vi "Motor Power Based on Vision.vi"() -> (1 "Right Motor Power":dbl, 3 "Left Motor Power":dbl)   [LabVIEW 2016]
uses:
  Robot Values.vi
  Vision Global.vi
  <vilib>/addons/control/pid/pid.llb/PID (DBL).vi
  <vilib>/addons/control/pid/NI_PID_pid.lvlib
panel:
  out "Vision Particles":dbl
  out "Done":bool
  in  "Vision PID Gains":T1={"proportional gain (Kc)"=0.2, "integral time (Ti, min)"=0.0, "derivative time (Td, min)"=0.0} {"derivative time (Td, min)" format="%.3f"; "integral time (Ti, min)" format="%.3f"; "proportional gain (Kc)" format="%.3f"}
  in  "Power Baseline":dbl=0.5
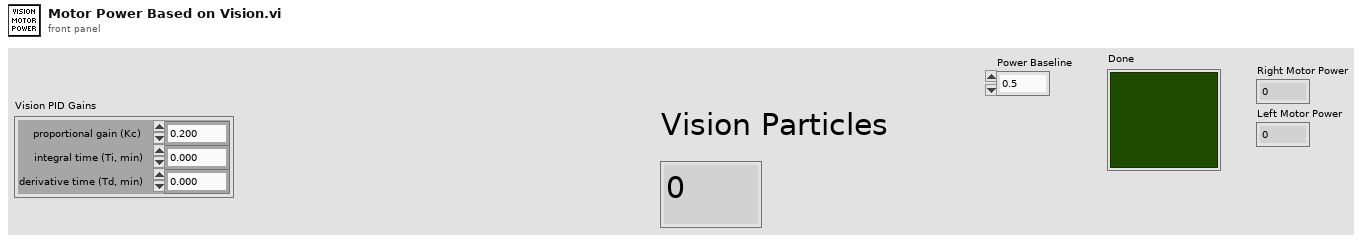
[diagram p1: front panel]
types:
  T1 = cluster{"proportional gain (Kc)":dbl, "integral time (Ti, min)":dbl, "derivative time (Td, min)":dbl}
  T2 = typedef "Robot Values.ctl" = cluster{"Robot Drive":cluster{"Left Motor Power":dbl, "Right Motor Power":dbl, "Left Encoder Value":dbl, "Right Encoder Value":dbl, "High Gear?":bool, "PTO?":bool}, "Sensors":cluster{"Gyro Angle":u16, "Recalibrate Gyro":bool, "Reset Gyro":bool, "Ultrasonic":dbl}, "Shooter":cluster{"Prep Wheels":bool, "Shoot":bool, "Left Shooter Wheel Speed":dbl, "Wheels Moving":bool, "Shooter Prepped":bool, "Shooter RPS SP":dbl, "Shooting?":bool, "Left Shooter Wheel Power":dbl, "Right Shooter Wheel Power":dbl, "Acquisition Conveyor Power":dbl, "Hopper Beater Bar Power":dbl, "Filtered Left Shooter Speed":dbl, "Acquisition Motor Power":dbl, "Joystick Add":dbl}, "Robot States":cluster{"Drive mode":string, "Alliance":T3, "Position":T4}, "Gear":cluster{"Ejection Active":bool}}
  T3 = typedef "WPI_DriverStationAllianceInfo.ctl" = enum16{"Red", "Blue", "Invalid"}
  T4 = typedef "WPI_DriverStationPositionInfo.ctl" = enum16{"1", "2", "3"}
  T5 = cluster{"Distance (ft)":dbl, "Score":dbl, "Normalized":cluster{"Center":cluster{dbl, dbl}, "Rectangle":cluster{"Numeric":dbl, "Numeric 2":dbl, "Numeric 3":dbl, "Numeric 5":dbl}}, "Pixels":cluster{"Center":cluster{dbl, dbl}, "Rectangle":cluster{"Numeric":dbl, "Numeric 2":dbl, "Numeric 3":dbl, "Numeric 5":dbl}}}
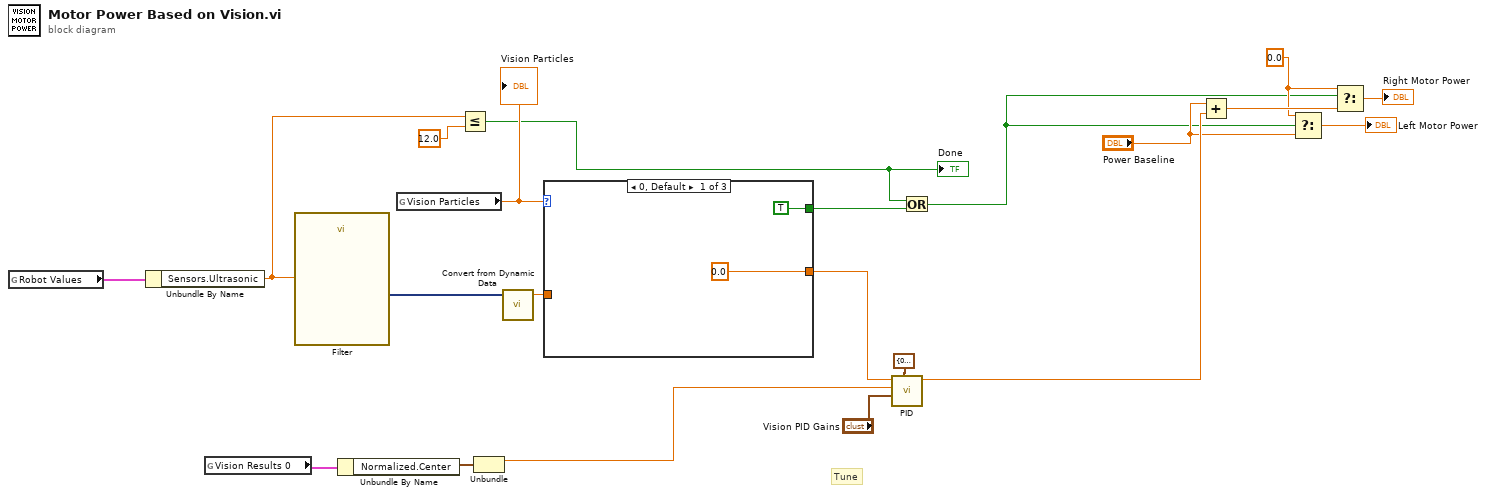
[diagram p0: block diagram]
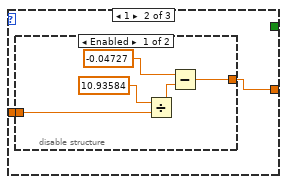
[diagram p2: hidden frame]
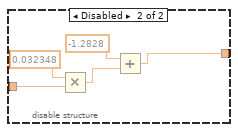
[diagram p3: hidden frame]
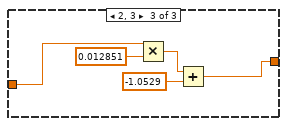
[diagram p4: hidden frame]
diagram:
  w16 = 0.0 ("t")
  # "Tune"
  n1 = global read "Robot Values.vi" "Robot Values"() -> (w12:T2)
  n2 = Unbundle By Name(w12) -> ("Sensors.Ultrasonic"=w7:dbl)
  n3 = global read "Vision Global.vi" "Vision Results 0"() -> (w21:T5)
  n4 = call "Filter"("Signal"=w7) -> ("Filtered Signal"=w8:dynamicdata)  [unwired: 9 in, 1 out]
  n5 = Unbundle By Name(w21) -> ("Normalized.Center"=w20:cluster{dbl, dbl})
  n6 = global read "Vision Global.vi" "Vision Particles"() -> (w9:dbl)
  "Vision Particles" <- w9
  n7 = Less Or Equal?(x=w7, y=12.0) -> (x <= y?=w3:bool)
  "Done" <- w3
  n8 = Unbundle(w20) -> (w15:dbl)  [unwired: 1 out]
  n9 = call "Convert from Dynamic Data"("Dynamic Data Type"=w8) -> ("Scalar"=w6:dbl)  [unwired: 3 in]
  n10 = case shown="0, Default" w9 {
    tunnel: w6 -> [_ w25 w37]
    tunnel: [0.0 w24 w36] -> w11
    tunnel: [TRUE _ _] -> w4
    frame 0, Default {
    }
    frame 1 {
      n11 = disable-structure shown="Enabled" {
        disable-tunnel: w25 -> [w29 w35]
        disable-tunnel: [w26 w31] -> w24
        frame Enabled {
          n12 = Divide(x=10.93584 ("y"), y=w29) -> (x/y=w27:dbl)
          n13 = Subtract(x=-0.04727 ("y"), y=w27) -> (x-y=w26:dbl)
        }
        frame Disabled {
          n14 = Multiply(x=0.032348, y=w35) -> (x*y=w33:dbl)
          n15 = Add(x=-1.2828, y=w33) -> (x+y=w31:dbl)
        }
      }
    }
    frame 2, 3 {
      n16 = Multiply(x=w37, y=0.012851) -> (x*y=w38:dbl)
      n17 = Add(x=w38, y=-1.0529) -> (x+y=w36:dbl)
    }
  }
  n18 = call-poly <vilib>:"PID.vi"("output range"=cluster{"output high":dbl, "output low":dbl} {"output high"=0.2, "output low"=-0.2}, "PID gains"="Vision PID Gains", "process variable"=w15, "setpoint"=w11) -> ("output"=w14:dbl)  [unwired: 6 in, 1 out]
  n19 = Or(x=w3, y=w4) -> (x .or. y?=w5:bool)
  n20 = Add(x="Power Baseline", y=w14) -> (x+y=w17:dbl)
  n21 = Select(t=w16, s=w5, f="Power Baseline") -> (s? t:f=→"Left Motor Power":dbl)
  n22 = Select(t=w16, s=w5, f=w17) -> (s? t:f=→"Right Motor Power":dbl)
